vi "首页.vi"() -> ()   [LabVIEW 2016]
uses:
  <vilib>/Utility/miscctls.llb/LVPointTypeDef.ctl
  <vilib>/Utility/sysdir.llb/System Directory Type.ctl
  <vilib>/addons/database/_DB Variant To Data/Database Variant To Data.xnode
  PLC/PLC.lvlib
  <vilib>/ptbypt/NI_PtbyPt.lvlib
panel:
  out "大项目框 17":T1(xcontrol)
  out "大项目框 16":T1(xcontrol)
  out "大项目框 15":T1(xcontrol)
  out "大项目框 14":T1(xcontrol)
  out "大项目框 13":T1(xcontrol)
  in  "左箭头":bool
  in  "右箭头":bool
  out "大项目框 12":T1(xcontrol)
  out "大项目框 11":T1(xcontrol)
  out "大项目框 10":T1(xcontrol)
  out "大项目框 9":T1(xcontrol)
  out "大项目框 8":T1(xcontrol)
  out "大项目框 7":T1(xcontrol)
  out "大项目框 6":T1(xcontrol)
  out "大项目框 5":T1(xcontrol)
  out "大项目框 4":T1(xcontrol)
  out "大项目框 3":T1(xcontrol)
  out "大项目框 2":T1(xcontrol)
  out "大项目框":T1(xcontrol)
  out "湿度":string="75.5 %"
  out "室温":string="25.8 ℃"
  # "室温:"
  # "湿度:"
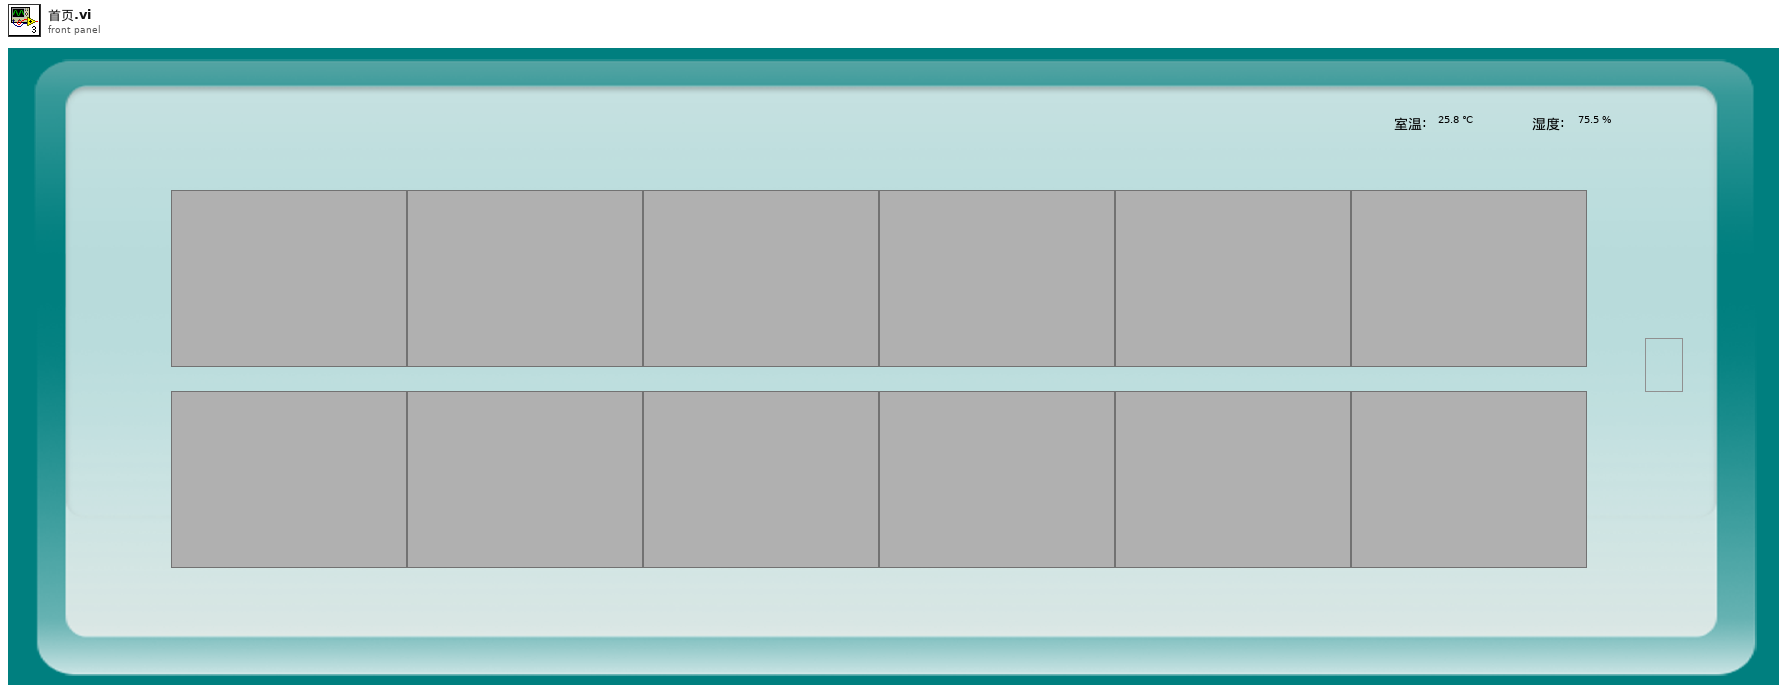
[diagram p1: front panel]
types:
  T1 = cluster{"中文项目名称":string, "英文项目名称":string, "单位":string, "浓度值":string}
  T2 = typedef "LVPointTypeDef.ctl" = cluster{"Horizontal":i16, "Vertical":i16}
  T3 = cluster{"AD0":sgl, "AD1":sgl, "AD2":sgl, "AD3":sgl, "AD4":sgl, "AD5":sgl}
  T4 = typedef "LVDateTimeRec.ctl" = cluster{"秒数的小数部分":dbl, "秒":i32, "分":i32, "时":i32, "日":i32, "月":i32, "年":i32, "天数（周）":i32, "天数（年）":i32, "DST":i32}
  T5 = cluster{"时间标识":timestamp, "监测值":sgl, "单位":string}
  T6 = cluster{"显示参数中文名":string, "显示参数英文名":string, "显示浓度":string, "显示单位":string}[]
  T7 = cluster{"显示参数中文名":string, "显示参数英文名":string, "显示浓度":string, "显示单位":string}
  T8 = typedef "System Directory Type.ctl" = i32
  T9 = cluster{"水温":bool, "pH":bool, "DO":bool, "Cond":bool, "Turb":bool, "氨氮":bool, "总磷":bool, "总氮":bool, "CODMn":bool, "CODCr":bool, "水位":bool, "流速":bool, "瞬时流量":bool, "室温":bool, "湿度":bool, "叶绿素a":bool, "藻密度":bool}
  T10 = cluster{"中文项目名称":string, "英文项目名称":string, "浓度值":string, "单位":string}
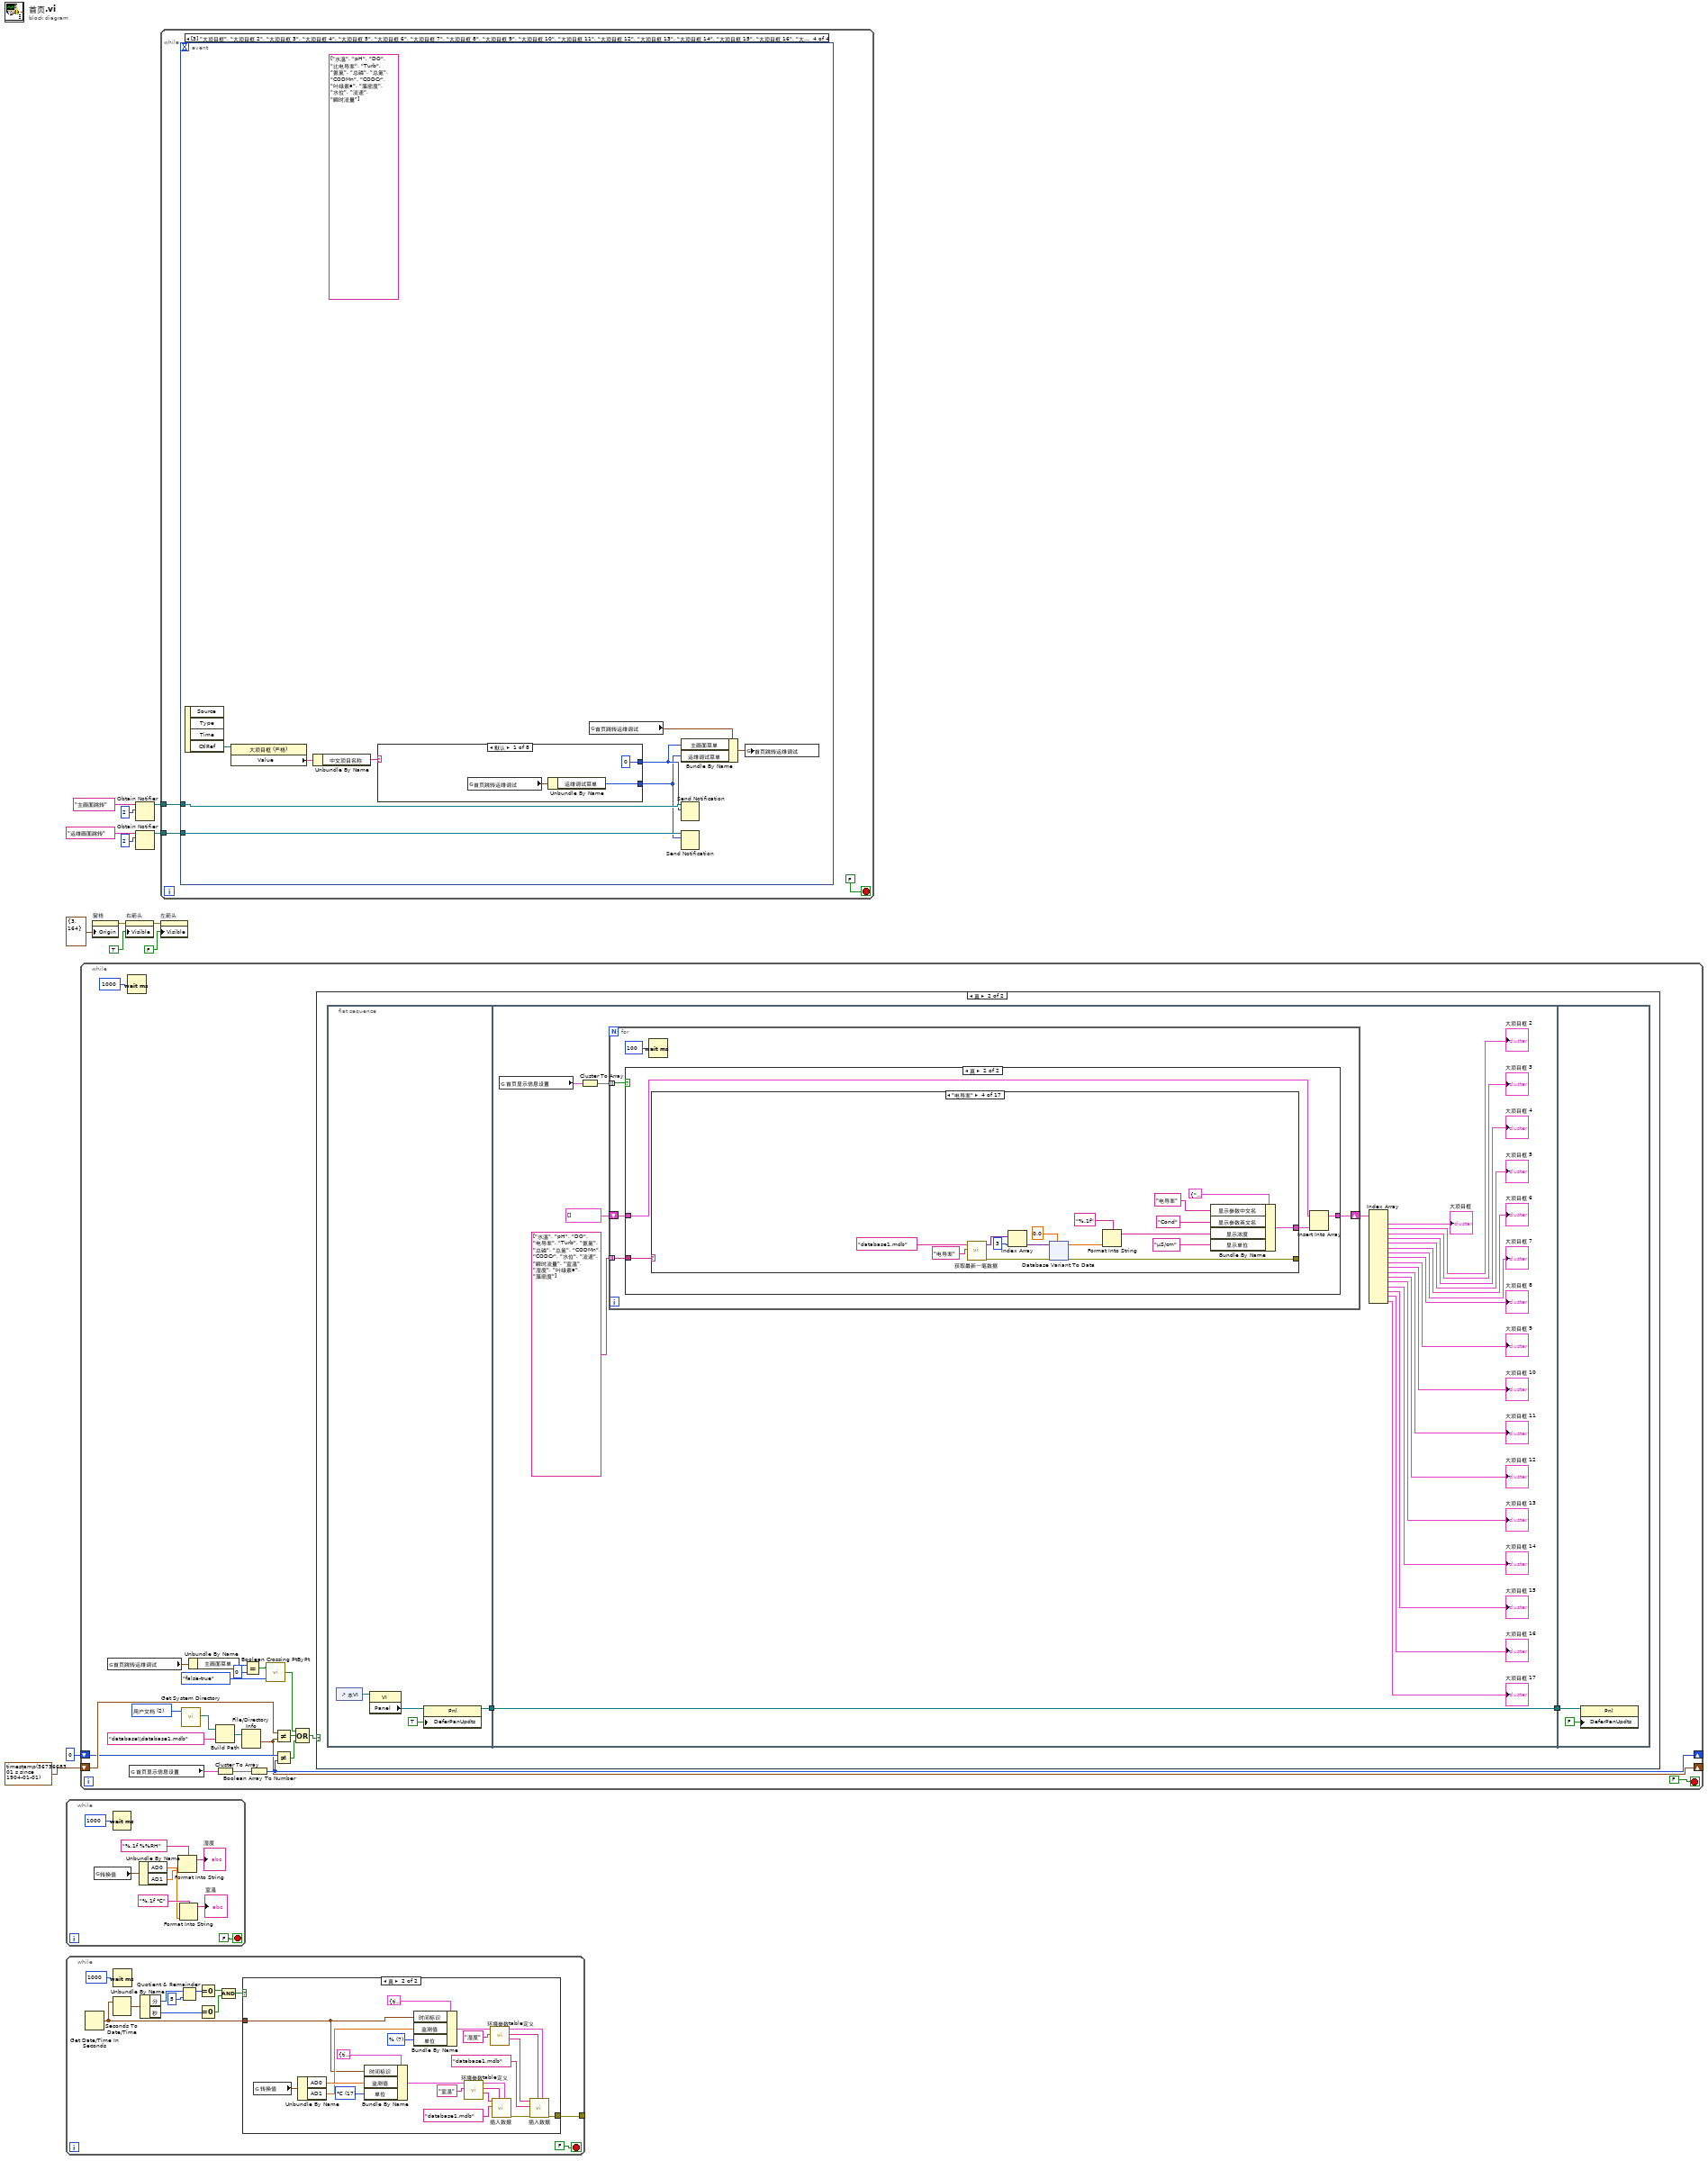
[diagram p0: block diagram]
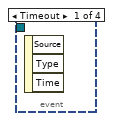
[diagram p3: hidden frame]
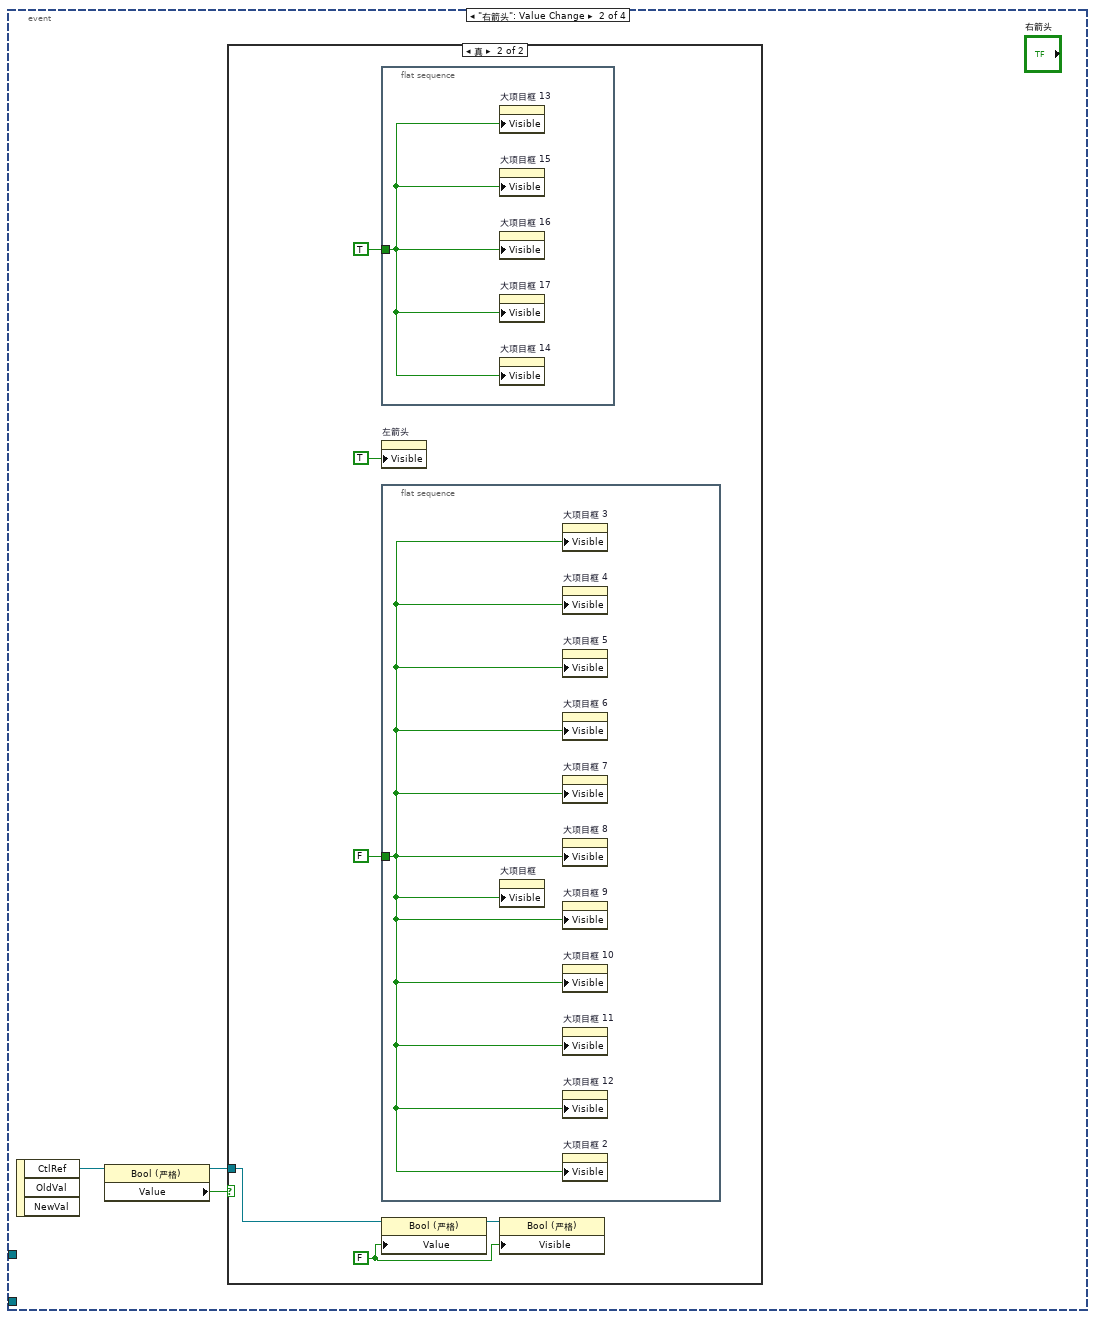
[diagram p4: hidden frame]
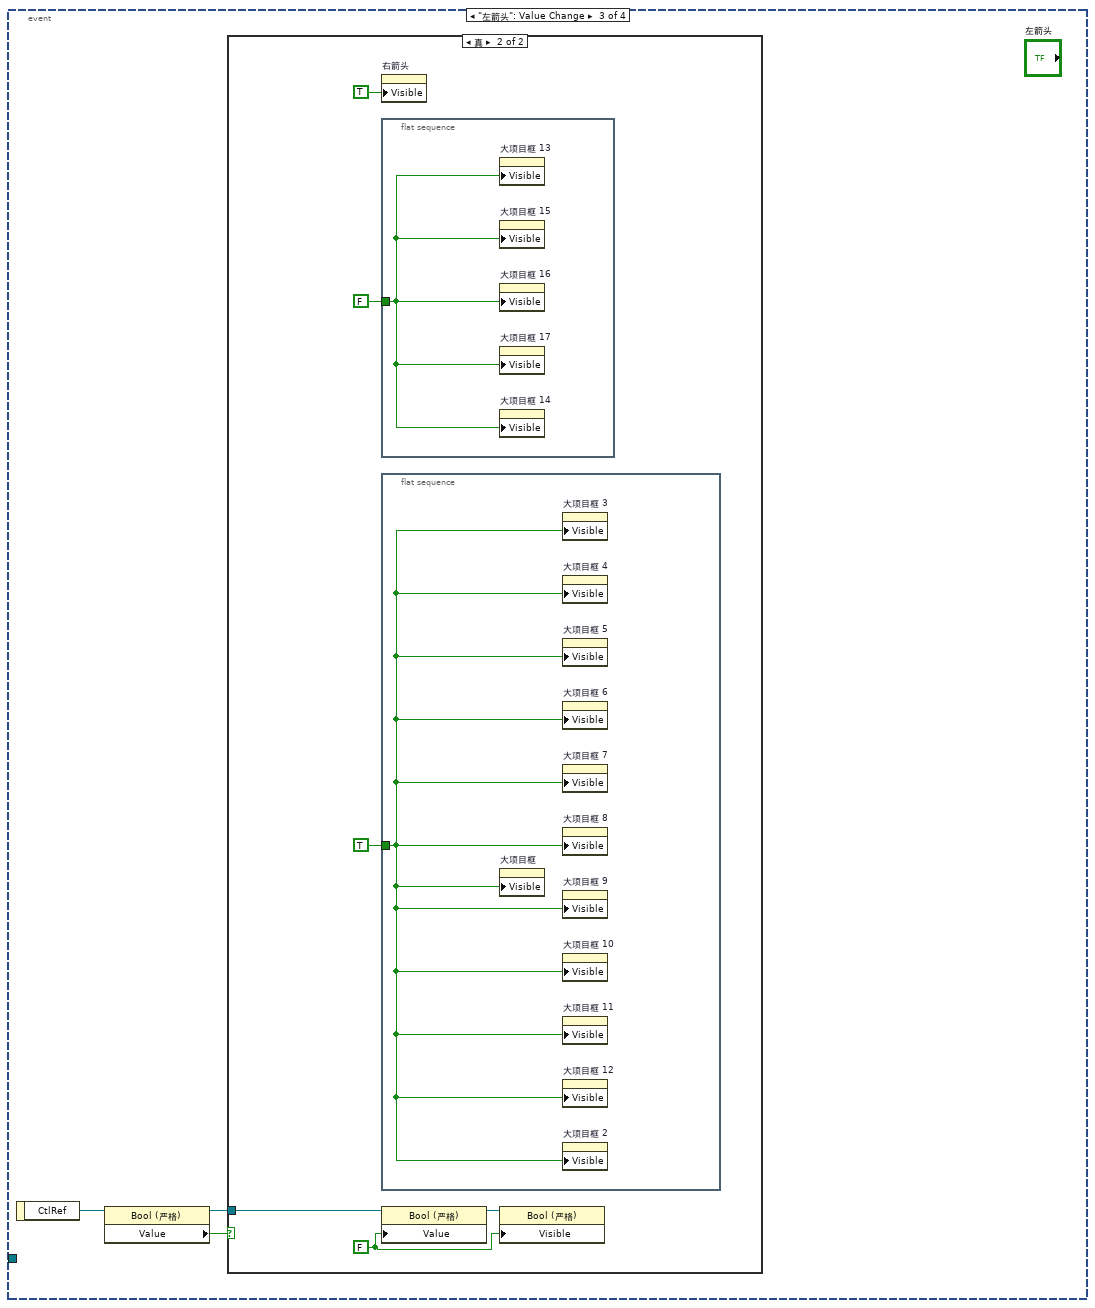
[diagram p6: hidden frame]
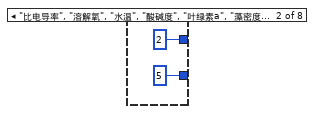
[diagram p8: hidden frame]
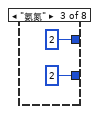
[diagram p9: hidden frame]
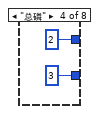
[diagram p10: hidden frame]
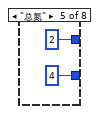
[diagram p11: hidden frame]
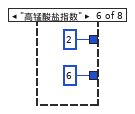
[diagram p12: hidden frame]
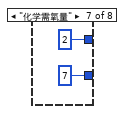
[diagram p13: hidden frame]
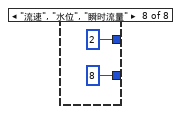
[diagram p14: hidden frame]
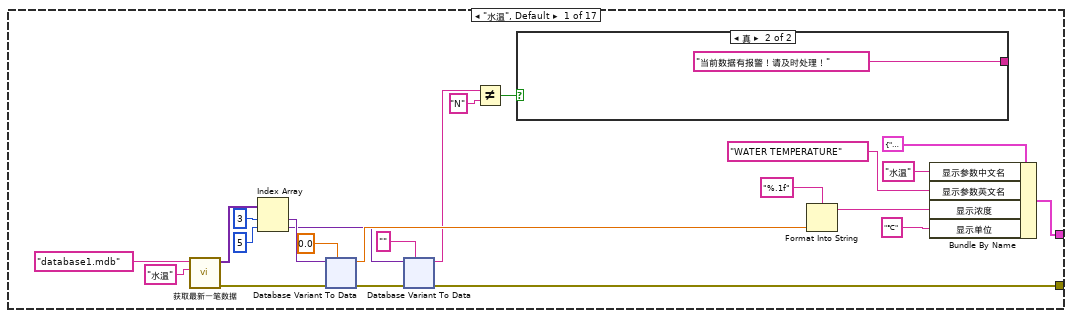
[diagram p17: hidden frame]
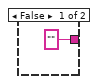
[diagram p18: hidden frame]
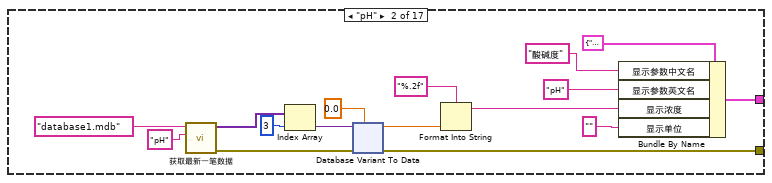
[diagram p19: hidden frame]
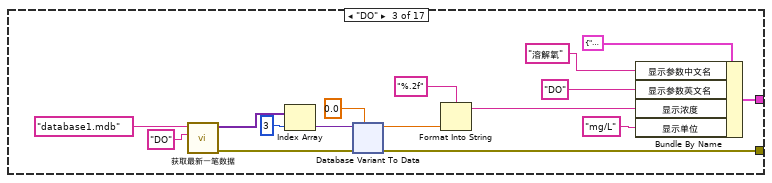
[diagram p20: hidden frame]
diagram:
  n1 = while {
    stop <- FALSE stop-if-true
    n2 = global read "采配水全局变量.vi" "转换值"() -> (w20:T3)
    n3 = Wait (ms)(milliseconds to wait=u32 1000 ("等待时间（毫秒）")) -> ()  [unwired: 1 out]
    n4 = Unbundle By Name(w20) -> ("AD0"=w15:sgl, "AD1"=w14:sgl)
    n5 = Format Into String(format string="%.1f %%RH" ("格式字符串"), w14) -> (resulting string=→"湿度":string)  [unwired: 2 in, 1 out]
    n6 = Format Into String(format string="%.1f ℃" ("格式字符串"), w15) -> (resulting string=→"室温":string)  [unwired: 2 in, 1 out]
  }
  n7 = while {
    tunnel: [w33] -> _
    stop <- FALSE stop-if-true
    n8 = Get Date/Time In Seconds() -> (seconds since 1Jan1904=w32:timestamp)
    n9 = Seconds To Date/Time(time stamp (now)=w32) -> (date time rec=w31:T4)  [unwired: 1 in]
    n10 = Wait (ms)(milliseconds to wait=u32 1000 ("等待时间（毫秒）")) -> ()  [unwired: 1 out]
    n11 = Unbundle By Name(w31) -> ("分"=w30:i32, "秒"=w28:i32)
    n12 = Quotient & Remainder(x=w30, y=5) -> (x-y*floor(x/y)=w27:i32)  [unwired: 1 out]
    n13 = Equal To 0?(x=w27) -> (x = 0?=w26:bool)
    n14 = Equal To 0?(x=w28) -> (x = 0?=w25:bool)
    n15 = Compound Arithmetic op=AND ("复合运算")(w26, w25) -> (w24:bool)
    n16 = case shown="真" w24 {
      tunnel: [_ w48] -> w33
      tunnel: w32 -> [_ w36]
      frame False {
      }
      frame True {
        w41 = u16 7 items=["ug/L", "mg/L", "ppm", "mg/m3", "cm", "ppb", "ug/m3", "%", "nmol/mol", "umol/mol", "MPN/L", "MPN/100ml", "ng/m3", "NTU", "无量纲", "ms/cm", "us/cm", "℃", "V"] ("单位")
        w45 = u16 17 items=["ug/L", "mg/L", "ppm", "mg/m3", "cm", "ppb", "ug/m3", "%", "nmol/mol", "umol/mol", "MPN/L", "MPN/100ml", "ng/m3", "NTU", "无量纲", "ms/cm", "us/cm", "℃", "V"] ("单位")
        n17 = global read "采配水全局变量.vi" "转换值"() -> (w56:T3)
        n18 = Unbundle By Name(w56) -> ("AD0"=w44:sgl, "AD1"=w42:sgl)
        n19 = Bundle By Name(cluster=cluster{"时间标识":timestamp, "监测值":sgl, "单位":u16} {"时间标识"=timestamp(0 s since 1904-01-01), "监测值"=0.0, "单位"=0} ("data"), "时间标识"=w36, "监测值"=w44, "单位"=w45) -> (w46:cluster{"时间标识":timestamp, "监测值":sgl, "单位":u16})
        n20 = Bundle By Name(cluster=cluster{"时间标识":timestamp, "监测值":sgl, "单位":u16} {"时间标识"=timestamp(0 s since 1904-01-01), "监测值"=0.0, "单位"=0} ("data"), "时间标识"=w36, "监测值"=w42, "单位"=w41) -> (w40:cluster{"时间标识":timestamp, "监测值":sgl, "单位":u16})
        n21 = call "环境参数table定义.vi"("table 输入"="室温", "data"=w46) -> ("table 输出"=w55:string, "columns"=w54:string[], "data输出"=w53:T5)  [unwired: 7 in]
        n22 = call "环境参数table定义.vi"("table 输入"="湿度", "data"=w40) -> ("table 输出"=w50:string, "columns"=w51:string[], "data输出"=w52:T5)  [unwired: 7 in]
        n23 = call "插入数据.vi"("data"=w53, "columns"=w54, "database"="database1.mdb" ("table 输入"), "table"=w55) -> ("error out"=w49:errorcluster)  [unwired: 7 in]
        n24 = call "插入数据.vi"("data"=w52, "columns"=w51, "error in (no error)"=w49, "database"="database1.mdb" ("table 输入"), "table"=w50) -> ("error out"=w48:errorcluster)  [unwired: 6 in]
      }
    }
  }
  n25 = while {
    shift-right: [w63] -> _
    shift-left: timestamp(3673668301 s since 1904-01-01) ("上次修改") -> [w72]
    shift-right: [w65] -> _
    shift-left: u32 0 ("数字") -> [w67]
    stop <- FALSE stop-if-true
    w75 = T8 2 items=["用户目录"=0, "用户桌面"=1, "用户文档"=2, "用户应用程序数据"=3, "用户设置"=4, "用户临时目录"=5, "公共文档"=6, "公共应用程序数据"=7, "公共设置"=8, "公共缓存"=13, "系统核心库"=9, "系统安装库"=10, "应用程序文件"=11, "启动盘根目录"=12] ("system directory type")
    n26 = global read "系统设置全局变量.vi" "首页跳转运维调试"() -> (w62:cluster{"主画面菜单":i32, "运维调试菜单":i32})
    n27 = Wait (ms)(milliseconds to wait=u32 1000 ("等待时间（毫秒）")) -> ()  [unwired: 1 out]
    n28 = global read "系统设置全局变量.vi" "首页显示信息设置"() -> (w69:T9)
    n29 = call <vilib>:"Get System Directory.vi"("system directory type"=w75) -> ("system directory"=w74:path)  [unwired: 10 in]
    n30 = Unbundle By Name(w62) -> ("主画面菜单"=w61:i32)
    n31 = Build Path(base path=w74, name or relative path="database\\database1.mdb" ("名称或相对路径")) -> (appended path=w64:path)
    n32 = Cluster To Array(cluster=w69) -> (array=w68:bool[])
    n33 = File/Directory Info(path=w64) -> (last mod=w63:timestamp)  [unwired: 1 in, 6 out]
    n34 = Equal?(x=w61, y=0) -> (x = y?=w59:bool)
    n35 = Boolean Array To Number(Boolean array=w68) -> (number=w65:u32)
    n36 = call <vilib>:"Boolean Crossing PtByPt.vi"("direction"=enum16{"either", "false-true", "true-false"}."false-true", "input"=w59) -> ("crossing"=w57:bool)  [unwired: 1 in]
    n37 = Not Equal?(x=w72, y=w63) -> (x != y?=w71:bool)
    n38 = Not Equal?(x=w67, y=w65) -> (x != y?=w66:bool)
    n39 = Compound Arithmetic op=OR ("复合运算")(w57, w71, w66) -> (w70:bool)
    n40 = case shown="真" w70 {
      frame False {
      }
      frame True {
        n41 = flat-sequence {
          tunnel: [w80] -> w78
          tunnel: [w84] -> w79
          tunnel: w78 -> [w84]
          tunnel: w79 -> [w777]
          frame #0 {
            n42 = control-ref of="本VI"() -> (w81:refnum<vi>)
            n43 = property class="VI"(reference=w81) -> ("Panel"=w82:refnum<vi>)  [unwired: 1 in, 2 out]
            n44 = property class="Pnl"(reference=w82, "DeferPanUpdts"=TRUE ("延迟前面板更新")) -> (reference out=w80:refnum<vi>)  [unwired: 1 in, 1 out]
          }
          frame #1 {
            n45 = global read "系统设置全局变量.vi" "首页显示信息设置"() -> (w86:T9)
            n46 = Cluster To Array(cluster=w86) -> (array=w85:bool[])
            n47 = for {
              tunnel: w85 -> [w111] mode=indexing
              tunnel: string[] ["水温", "pH", "DO", "电导率", "Turb", "氨氮", "总磷", "总氮", "CODMn", "CODCr", "水位", "流速", "瞬时流量", "室温", "湿度", "叶绿素a", "藻密度"] -> [w110] mode=indexing
              shift-right: [w108] -> w106
              shift-left: T6 [] -> [w109]
              n48 = case shown="真" w111 {
                tunnel: w110 -> [_ w116]
                tunnel: w109 -> [w112 w115]
                tunnel: [w112 w114] -> w108
                frame False {
                }
                frame True {
                  n49 = case shown="\"电导率\"" w116 {
                    tunnel: [w125 w217 w265 w313 w361 w409 w457 w505 w553 w601 w639 w687 w737 w745 w750 w760 w769] -> w113
                    tunnel: [w117 w206 w254 w302 w350 w398 w446 w494 w542 w590 w638 w686 _ _ _ _ _] -> _
                    frame "水温", Default {
                      n50 = call "获取最新一笔数据.vi"("table"="水温", "database"="database1.mdb" ("名称或相对路径")) -> ("error out"=w126:errorcluster, "子数组"=w132:variant[])  [unwired: 8 in]
                      n51 = Index Array(array=w132, index #1=3 ("索引"), index #2=5 ("索引")) -> (element #1=w130:variant, element #2=w122:variant)
                      n52 = xnode "Database Variant To Data"("database variant"=w130, "error in (no error)"=w126, "type"=0.0) -> ("data"=w127:dbl, "error out"=w118:errorcluster)
                      n53 = xnode "Database Variant To Data"("database variant"=w122, "error in (no error)"=w118, "type"="") -> ("data"=w121:string, "error out"=w117:errorcluster)
                      n54 = Not Equal?(x=w121, y="N") -> (x != y?=w119:bool)
                      n55 = case shown="真" w119 {
                        tunnel: ["" "当前数据有报警！请及时处理！" ("y")] -> _
                        frame False {
                        }
                        frame True {
                        }
                      }
                      n56 = Format Into String(format string="%.1f" ("格式字符串"), w127) -> (resulting string=w134:string)  [unwired: 2 in, 1 out]
                      n57 = Bundle By Name(cluster=T7 {"显示参数中文名"="", "显示参数英文名"="", "显示浓度"="", "显示单位"=""} ("元素"), "显示参数中文名"="水温", "显示参数英文名"="WATER TEMPERATURE", "显示浓度"=w134, "显示单位"="℃") -> (w125:T7)
                    }
                    frame "pH" {
                      n58 = call "获取最新一笔数据.vi"("table"="pH", "database"="database1.mdb" ("名称或相对路径")) -> ("error out"=w207:errorcluster, "子数组"=w213:variant[])  [unwired: 8 in]
                      n59 = Index Array(array=w213, index=3 ("索引")) -> (element=w211:variant)
                      n60 = xnode "Database Variant To Data"("database variant"=w211, "error in (no error)"=w207, "type"=0.0) -> ("data"=w208:dbl, "error out"=w206:errorcluster)
                      n61 = Format Into String(format string="%.2f" ("格式字符串"), w208) -> (resulting string=w215:string)  [unwired: 2 in, 1 out]
                      n62 = Bundle By Name(cluster=T7 {"显示参数中文名"="", "显示参数英文名"="", "显示浓度"="", "显示单位"=""} ("元素"), "显示参数中文名"="酸碱度", "显示参数英文名"="pH", "显示浓度"=w215, "显示单位"="") -> (w217:T7)
                    }
                    frame "DO" {
                      n63 = call "获取最新一笔数据.vi"("table"="DO", "database"="database1.mdb" ("名称或相对路径")) -> ("error out"=w255:errorcluster, "子数组"=w261:variant[])  [unwired: 8 in]
                      n64 = Index Array(array=w261, index=3 ("索引")) -> (element=w259:variant)
                      n65 = xnode "Database Variant To Data"("database variant"=w259, "error in (no error)"=w255, "type"=0.0) -> ("data"=w256:dbl, "error out"=w254:errorcluster)
                      n66 = Format Into String(format string="%.2f" ("格式字符串"), w256) -> (resulting string=w263:string)  [unwired: 2 in, 1 out]
                      n67 = Bundle By Name(cluster=T7 {"显示参数中文名"="", "显示参数英文名"="", "显示浓度"="", "显示单位"=""} ("元素"), "显示参数中文名"="溶解氧", "显示参数英文名"="DO", "显示浓度"=w263, "显示单位"="mg/L") -> (w265:T7)
                    }
                    frame "电导率" {
                      n68 = call "获取最新一笔数据.vi"("table"="电导率", "database"="database1.mdb" ("名称或相对路径")) -> ("error out"=w303:errorcluster, "子数组"=w309:variant[])  [unwired: 8 in]
                      n69 = Index Array(array=w309, index=3 ("索引")) -> (element=w307:variant)
                      n70 = xnode "Database Variant To Data"("database variant"=w307, "error in (no error)"=w303, "type"=0.0) -> ("data"=w304:dbl, "error out"=w302:errorcluster)
                      n71 = Format Into String(format string="%.1f" ("格式字符串"), w304) -> (resulting string=w311:string)  [unwired: 2 in, 1 out]
                      n72 = Bundle By Name(cluster=T7 {"显示参数中文名"="", "显示参数英文名"="", "显示浓度"="", "显示单位"=""} ("元素"), "显示参数中文名"="电导率", "显示参数英文名"="Cond", "显示浓度"=w311, "显示单位"="μS/cm") -> (w313:T7)
                    }
                    frame "Turb" {
                      n73 = call "获取最新一笔数据.vi"("table"="浊度", "database"="database1.mdb" ("名称或相对路径")) -> ("error out"=w351:errorcluster, "子数组"=w357:variant[])  [unwired: 8 in]
                      n74 = Index Array(array=w357, index=3 ("索引")) -> (element=w355:variant)
                      n75 = xnode "Database Variant To Data"("database variant"=w355, "error in (no error)"=w351, "type"=0.0) -> ("data"=w352:dbl, "error out"=w350:errorcluster)
                      n76 = Format Into String(format string="%.1f" ("格式字符串"), w352) -> (resulting string=w359:string)  [unwired: 2 in, 1 out]
                      n77 = Bundle By Name(cluster=T7 {"显示参数中文名"="", "显示参数英文名"="", "显示浓度"="", "显示单位"=""} ("元素"), "显示参数中文名"="浊度", "显示参数英文名"="Turb", "显示浓度"=w359, "显示单位"="NTU") -> (w361:T7)
                    }
                    frame "氨氮" {
                      n78 = call "获取最新一笔数据.vi"("table"="氨氮", "database"="database1.mdb" ("名称或相对路径")) -> ("error out"=w399:errorcluster, "子数组"=w405:variant[])  [unwired: 8 in]
                      n79 = Index Array(array=w405, index=3 ("索引")) -> (element=w403:variant)
                      n80 = xnode "Database Variant To Data"("database variant"=w403, "error in (no error)"=w399, "type"=0.0) -> ("data"=w400:dbl, "error out"=w398:errorcluster)
                      n81 = Format Into String(format string="%.3f" ("格式字符串"), w400) -> (resulting string=w407:string)  [unwired: 2 in, 1 out]
                      n82 = Bundle By Name(cluster=T7 {"显示参数中文名"="", "显示参数英文名"="", "显示浓度"="", "显示单位"=""} ("元素"), "显示参数中文名"="氨氮", "显示参数英文名"="NPA", "显示浓度"=w407, "显示单位"="mg/L") -> (w409:T7)
                    }
                    frame "总磷" {
                      n83 = call "获取最新一笔数据.vi"("table"="总磷", "database"="database1.mdb" ("名称或相对路径")) -> ("error out"=w447:errorcluster, "子数组"=w453:variant[])  [unwired: 8 in]
                      n84 = Index Array(array=w453, index=3 ("索引")) -> (element=w451:variant)
                      n85 = xnode "Database Variant To Data"("database variant"=w451, "error in (no error)"=w447, "type"=0.0) -> ("data"=w448:dbl, "error out"=w446:errorcluster)
                      n86 = Format Into String(format string="%.3f" ("格式字符串"), w448) -> (resulting string=w455:string)  [unwired: 2 in, 1 out]
                      n87 = Bundle By Name(cluster=T7 {"显示参数中文名"="", "显示参数英文名"="", "显示浓度"="", "显示单位"=""} ("元素"), "显示参数中文名"="总磷", "显示参数英文名"="TP", "显示浓度"=w455, "显示单位"="mg/L") -> (w457:T7)
                    }
                    frame "总氮" {
                      n88 = call "获取最新一笔数据.vi"("table"="总氮", "database"="database1.mdb" ("名称或相对路径")) -> ("error out"=w495:errorcluster, "子数组"=w501:variant[])  [unwired: 8 in]
                      n89 = Index Array(array=w501, index=3 ("索引")) -> (element=w499:variant)
                      n90 = xnode "Database Variant To Data"("database variant"=w499, "error in (no error)"=w495, "type"=0.0) -> ("data"=w496:dbl, "error out"=w494:errorcluster)
                      n91 = Format Into String(format string="%.2f" ("格式字符串"), w496) -> (resulting string=w503:string)  [unwired: 2 in, 1 out]
                      n92 = Bundle By Name(cluster=T7 {"显示参数中文名"="", "显示参数英文名"="", "显示浓度"="", "显示单位"=""} ("元素"), "显示参数中文名"="总氮", "显示参数英文名"="TN", "显示浓度"=w503, "显示单位"="mg/L") -> (w505:T7)
                    }
                    frame "CODMn" {
                      n93 = call "获取最新一笔数据.vi"("table"="CODmn", "database"="database1.mdb" ("名称或相对路径")) -> ("error out"=w543:errorcluster, "子数组"=w549:variant[])  [unwired: 8 in]
                      n94 = Index Array(array=w549, index=3 ("索引")) -> (element=w547:variant)
                      n95 = xnode "Database Variant To Data"("database variant"=w547, "error in (no error)"=w543, "type"=0.0) -> ("data"=w544:dbl, "error out"=w542:errorcluster)
                      n96 = Format Into String(format string="%.2f" ("格式字符串"), w544) -> (resulting string=w551:string)  [unwired: 2 in, 1 out]
                      n97 = Bundle By Name(cluster=T7 {"显示参数中文名"="", "显示参数英文名"="", "显示浓度"="", "显示单位"=""} ("元素"), "显示参数中文名"="高锰酸盐指数", "显示参数英文名"="CODmn", "显示浓度"=w551, "显示单位"="mg/L") -> (w553:T7)
                    }
                    frame "CODCr" {
                      n98 = call "获取最新一笔数据.vi"("table"="CODCr", "database"="database1.mdb" ("名称或相对路径")) -> ("error out"=w591:errorcluster, "子数组"=w597:variant[])  [unwired: 8 in]
                      n99 = Index Array(array=w597, index=3 ("索引")) -> (element=w595:variant)
                      n100 = xnode "Database Variant To Data"("database variant"=w595, "error in (no error)"=w591, "type"=0.0) -> ("data"=w592:dbl, "error out"=w590:errorcluster)
                      n101 = Format Into String(format string="%.2f" ("格式字符串"), w592) -> (resulting string=w599:string)  [unwired: 2 in, 1 out]
                      n102 = Bundle By Name(cluster=T7 {"显示参数中文名"="", "显示参数英文名"="", "显示浓度"="", "显示单位"=""} ("元素"), "显示参数中文名"="化学需氧量", "显示参数英文名"="CODCr", "显示浓度"=w599, "显示单位"="mg/L") -> (w601:T7)
                    }
                    frame "叶绿素a" {
                      n103 = call "获取最新一笔数据.vi"("table"="叶绿素a", "database"="database1.mdb" ("名称或相对路径")) -> ("error out"=w640:errorcluster, "子数组"=w646:variant[])  [unwired: 8 in]
                      n104 = Index Array(array=w646, index=3 ("索引")) -> (element=w644:variant)
                      n105 = xnode "Database Variant To Data"("database variant"=w644, "error in (no error)"=w640, "type"=0.0) -> ("data"=w641:dbl, "error out"=w638:errorcluster)
                      n106 = Format Into String(format string="%.2f" ("格式字符串"), w641) -> (resulting string=w648:string)  [unwired: 2 in, 1 out]
                      n107 = Bundle By Name(cluster=T7 {"显示参数中文名"="", "显示参数英文名"="", "显示浓度"="", "显示单位"=""} ("元素"), "显示参数中文名"="叶绿素a", "显示参数英文名"="Chla", "显示浓度"=w648, "显示单位"="μg/L") -> (w639:T7)
                    }
                    frame "藻密度" {
                      n108 = call "获取最新一笔数据.vi"("table"="藻密度", "database"="database1.mdb" ("名称或相对路径")) -> ("error out"=w688:errorcluster, "子数组"=w694:variant[])  [unwired: 8 in]
                      n109 = Index Array(array=w694, index=3 ("索引")) -> (element=w692:variant)
                      n110 = xnode "Database Variant To Data"("database variant"=w692, "error in (no error)"=w688, "type"=0.0) -> ("data"=w689:dbl, "error out"=w686:errorcluster)
                      n111 = Format Into String(format string="%.2f" ("格式字符串"), w689) -> (resulting string=w696:string)  [unwired: 2 in, 1 out]
                      n112 = Bundle By Name(cluster=T7 {"显示参数中文名"="", "显示参数英文名"="", "显示浓度"="", "显示单位"=""} ("元素"), "显示参数中文名"="藻密度", "显示参数英文名"="Algal", "显示浓度"=w696, "显示单位"="cells/mL") -> (w687:T7)
                    }
                    frame "水位" {
                      n113 = global read "流量计全局变量.vi" "水位"() -> (w734:dbl)
                      n114 = Format Into String(format string="%.2f" ("格式字符串"), w734) -> (resulting string=w735:string)  [unwired: 2 in, 1 out]
                      n115 = Bundle By Name(cluster=T7 {"显示参数中文名"="", "显示参数英文名"="", "显示浓度"="", "显示单位"=""} ("元素"), "显示参数中文名"="水位", "显示参数英文名"="WaterLevel", "显示浓度"=w735, "显示单位"="m") -> (w737:T7)
                    }
                    frame "流速" {
                      n116 = global read "流量计全局变量.vi" "瞬时流速"() -> (w742:dbl)
                      n117 = Format Into String(format string="%.2f" ("格式字符串"), w742) -> (resulting string=w743:string)  [unwired: 2 in, 1 out]
                      n118 = Bundle By Name(cluster=T7 {"显示参数中文名"="", "显示参数英文名"="", "显示浓度"="", "显示单位"=""} ("元素"), "显示参数中文名"="流速", "显示参数英文名"="FlowRate", "显示浓度"=w743, "显示单位"="m/s") -> (w745:T7)
                    }
                    frame "瞬时流量" {
                      n119 = global read "流量计全局变量.vi" "瞬时流量"() -> (w751:dbl)
                      n120 = Format Into String(format string="%.2f" ("格式字符串"), w751) -> (resulting string=w752:string)  [unwired: 2 in, 1 out]
                      n121 = Bundle By Name(cluster=T7 {"显示参数中文名"="", "显示参数英文名"="", "显示浓度"="", "显示单位"=""} ("元素"), "显示参数中文名"="瞬时流量", "显示参数英文名"="InstantaneousFlow", "显示浓度"=w752, "显示单位"="m3/s") -> (w750:T7)
                    }
                    frame "室温" {
                      n122 = global read "采配水全局变量.vi" "转换值"() -> (w759:T3)
                      n123 = Unbundle By Name(w759) -> ("AD0"=w758:sgl)
                      n124 = Format Into String(format string="%.2f" ("格式字符串"), w758) -> (resulting string=w761:string)  [unwired: 2 in, 1 out]
                      n125 = Bundle By Name(cluster=T7 {"显示参数中文名"="", "显示参数英文名"="", "显示浓度"="", "显示单位"=""} ("元素"), "显示参数中文名"="室温", "显示参数英文名"="Room Temperature ", "显示浓度"=w761, "显示单位"="℃") -> (w760:T7)
                    }
                    frame "湿度" {
                      n126 = global read "采配水全局变量.vi" "转换值"() -> (w768:T3)
                      n127 = Unbundle By Name(w768) -> ("AD1"=w767:sgl)
                      n128 = Format Into String(format string="%.2f" ("格式字符串"), w767) -> (resulting string=w770:string)  [unwired: 2 in, 1 out]
                      n129 = Bundle By Name(cluster=T7 {"显示参数中文名"="", "显示参数英文名"="", "显示浓度"="", "显示单位"=""} ("元素"), "显示参数中文名"="相对湿度", "显示参数英文名"="Relative Humidity", "显示浓度"=w770, "显示单位"="%RH") -> (w769:T7)
                    }
                  }
                  n130 = Insert Into Array(array=w115, new element=w113) -> (w114:T6)  [unwired: 1 in]
                }
              }
              n131 = Wait (ms)(milliseconds to wait=u32 100 ("等待时间（毫秒）")) -> ()  [unwired: 1 out]
            }
            n132 = Index Array(array=w106) -> (element #1=→"大项目框":T7, element #2=→"大项目框 2":T7, element #3=→"大项目框 3":T7, element #4=→"大项目框 4":T7, element #5=→"大项目框 5":T7, element #6=→"大项目框 6":T7, element #7=→"大项目框 7":T7, element #8=→"大项目框 8":T7, element #9=→"大项目框 9":T7, element #10=→"大项目框 10":T7, element #11=→"大项目框 11":T7, element #12=→"大项目框 12":T7, element #13=→"大项目框 13":T7, element #14=→"大项目框 14":T7, element #15=→"大项目框 15":T7, element #16=→"大项目框 16":T7, element #17=→"大项目框 17":T7)  [unwired: 17 in]
          }
          frame #2 {
            n133 = property class="Pnl"(reference=w777, "DeferPanUpdts"=FALSE ("延迟前面板更新")) -> ()  [unwired: 1 in, 2 out]
          }
        }
      }
    }
  }
  n134 = property on="窗格" class="Pane"("Origin"=T2 {"Horizontal"=3, "Vertical"=164} ("原点")) -> (error out=w10:errorcluster)  [unwired: 2 in, 1 out]
  n135 = property on="右箭头" class="Bool (严格)"(error in=w10, "Visible"=TRUE ("可见")) -> (error out=w9:errorcluster)  [unwired: 1 in, 1 out]
  n136 = Obtain Notifier(name (unnamed)="主画面跳转" ("名称（未命名）"), notification data type=2 ("主画面菜单")) -> (notifier out=w8:refnum<notifier>)  [unwired: 2 in, 2 out]
  n137 = Obtain Notifier(name (unnamed)="运维画面跳转" ("名称（未命名）"), notification data type=2 ("主画面菜单")) -> (notifier out=w3:refnum<notifier>)  [unwired: 2 in, 2 out]
  n138 = property on="左箭头" class="Bool (严格)"(error in=w9, "Visible"=FALSE ("可见")) -> ()  [unwired: 1 in, 2 out]
  n139 = while {
    tunnel: w8 -> [w779]
    tunnel: w3 -> [w778]
    stop <- FALSE stop-if-true
    n140 = event shown="[3] \"大项目框\", \"大项目框 2\", \"大项目框 3\", \"大项目框 4\", \"大项目框 5\", \"大项目框 6\", \"大项目框 7\", \"大项目框 8\", \"大项目框 9\", \"大项目框 10\", \"大项目框 11\", \"大项目框 12\", \"大项目框 13\", \"大项目框 14\", \"大项目框 15\", \"大项目框 16\", \"大项目框 17\": 鼠标按下" {
      selector: _ -> [_ _ _ _]
      dyn-events: _ -> [_ _ _ _]
      timeout: _ -> [_ _ _ _]
      tunnel: w779 -> [_ _ _ w807]
      tunnel: w778 -> [_ _ _ w804]
      event Timeout {
        n141 = event-data() -> ()  [unwired: 1 in, 3 out]
      }
      event "右箭头": Value Change {
        n142 = event-data() -> ("CtlRef"=w783:refnum<vi>)  [unwired: 1 in, 2 out]
        n143 = property class="Bool (严格)"(reference=w783) -> (reference out=w781:refnum<vi>, "Value"=w782:bool)  [unwired: 1 in, 1 out]
        n144 = case shown="真" w782 {
          tunnel: w781 -> [_ w789]
          frame False {
          }
          frame True {
            w788 = FALSE ("值")
            n145 = flat-sequence {
              tunnel: TRUE ("可见") -> [w790]
              frame #0 {
                n146 = property on="大项目框 13" class="大项目框 (严格)"("Visible"=w790) -> ()  [unwired: 2 in, 2 out]
                n147 = property on="大项目框 15" class="大项目框 (严格)"("Visible"=w790) -> ()  [unwired: 2 in, 2 out]
                n148 = property on="大项目框 16" class="大项目框 (严格)"("Visible"=w790) -> ()  [unwired: 2 in, 2 out]
                n149 = property on="大项目框 17" class="大项目框 (严格)"("Visible"=w790) -> ()  [unwired: 2 in, 2 out]
                n150 = property on="大项目框 14" class="大项目框 (严格)"("Visible"=w790) -> ()  [unwired: 2 in, 2 out]
              }
            }
            n151 = property on="左箭头" class="Bool (严格)"("Visible"=TRUE ("可见")) -> ()  [unwired: 2 in, 2 out]
            n152 = flat-sequence {
              tunnel: FALSE ("可见") -> [w791]
              frame #0 {
                n153 = property on="大项目框" class="大项目框 (严格)"("Visible"=w791) -> ()  [unwired: 2 in, 2 out]
                n154 = property on="大项目框 3" class="大项目框 (严格)"("Visible"=w791) -> ()  [unwired: 2 in, 2 out]
                n155 = property on="大项目框 4" class="大项目框 (严格)"("Visible"=w791) -> ()  [unwired: 2 in, 2 out]
                n156 = property on="大项目框 5" class="大项目框 (严格)"("Visible"=w791) -> ()  [unwired: 2 in, 2 out]
                n157 = property on="大项目框 6" class="大项目框 (严格)"("Visible"=w791) -> ()  [unwired: 2 in, 2 out]
                n158 = property on="大项目框 7" class="大项目框 (严格)"("Visible"=w791) -> ()  [unwired: 2 in, 2 out]
                n159 = property on="大项目框 8" class="大项目框 (严格)"("Visible"=w791) -> ()  [unwired: 2 in, 2 out]
                n160 = property on="大项目框 9" class="大项目框 (严格)"("Visible"=w791) -> ()  [unwired: 2 in, 2 out]
                n161 = property on="大项目框 10" class="大项目框 (严格)"("Visible"=w791) -> ()  [unwired: 2 in, 2 out]
                n162 = property on="大项目框 11" class="大项目框 (严格)"("Visible"=w791) -> ()  [unwired: 2 in, 2 out]
                n163 = property on="大项目框 12" class="大项目框 (严格)"("Visible"=w791) -> ()  [unwired: 2 in, 2 out]
                n164 = property on="大项目框 2" class="大项目框 (严格)"("Visible"=w791) -> ()  [unwired: 2 in, 2 out]
              }
            }
            n165 = property class="Bool (严格)"(reference=w789, "Value"=w788) -> (reference out=w787:refnum<vi>)  [unwired: 1 in, 1 out]
            n166 = property class="Bool (严格)"(reference=w787, "Visible"=w788) -> ()  [unwired: 1 in, 2 out]
          }
        }
      }
      event "左箭头": Value Change {
        n167 = event-data() -> ("CtlRef"=w794:refnum<vi>)  [unwired: 1 in]
        n168 = property class="Bool (严格)"(reference=w794) -> (reference out=w792:refnum<vi>, "Value"=w793:bool)  [unwired: 1 in, 1 out]
        n169 = case shown="真" w793 {
          tunnel: w792 -> [_ w800]
          frame False {
          }
          frame True {
            w799 = FALSE ("值")
            n170 = property on="右箭头" class="Bool (严格)"("Visible"=TRUE ("可见")) -> ()  [unwired: 2 in, 2 out]
            n171 = flat-sequence {
              tunnel: FALSE ("可见") -> [w801]
              frame #0 {
                n172 = property on="大项目框 13" class="大项目框 (严格)"("Visible"=w801) -> ()  [unwired: 2 in, 2 out]
                n173 = property on="大项目框 15" class="大项目框 (严格)"("Visible"=w801) -> ()  [unwired: 2 in, 2 out]
                n174 = property on="大项目框 16" class="大项目框 (严格)"("Visible"=w801) -> ()  [unwired: 2 in, 2 out]
                n175 = property on="大项目框 17" class="大项目框 (严格)"("Visible"=w801) -> ()  [unwired: 2 in, 2 out]
                n176 = property on="大项目框 14" class="大项目框 (严格)"("Visible"=w801) -> ()  [unwired: 2 in, 2 out]
              }
            }
            n177 = flat-sequence {
              tunnel: TRUE ("可见") -> [w802]
              frame #0 {
                n178 = property on="大项目框" class="大项目框 (严格)"("Visible"=w802) -> ()  [unwired: 2 in, 2 out]
                n179 = property on="大项目框 3" class="大项目框 (严格)"("Visible"=w802) -> ()  [unwired: 2 in, 2 out]
                n180 = property on="大项目框 4" class="大项目框 (严格)"("Visible"=w802) -> ()  [unwired: 2 in, 2 out]
                n181 = property on="大项目框 5" class="大项目框 (严格)"("Visible"=w802) -> ()  [unwired: 2 in, 2 out]
                n182 = property on="大项目框 6" class="大项目框 (严格)"("Visible"=w802) -> ()  [unwired: 2 in, 2 out]
                n183 = property on="大项目框 7" class="大项目框 (严格)"("Visible"=w802) -> ()  [unwired: 2 in, 2 out]
                n184 = property on="大项目框 8" class="大项目框 (严格)"("Visible"=w802) -> ()  [unwired: 2 in, 2 out]
                n185 = property on="大项目框 9" class="大项目框 (严格)"("Visible"=w802) -> ()  [unwired: 2 in, 2 out]
                n186 = property on="大项目框 10" class="大项目框 (严格)"("Visible"=w802) -> ()  [unwired: 2 in, 2 out]
                n187 = property on="大项目框 11" class="大项目框 (严格)"("Visible"=w802) -> ()  [unwired: 2 in, 2 out]
                n188 = property on="大项目框 12" class="大项目框 (严格)"("Visible"=w802) -> ()  [unwired: 2 in, 2 out]
                n189 = property on="大项目框 2" class="大项目框 (严格)"("Visible"=w802) -> ()  [unwired: 2 in, 2 out]
              }
            }
            n190 = property class="Bool (严格)"(reference=w800, "Value"=w799) -> (reference out=w798:refnum<vi>)  [unwired: 1 in, 1 out]
            n191 = property class="Bool (严格)"(reference=w798, "Visible"=w799) -> ()  [unwired: 1 in, 2 out]
          }
        }
      }
      event "大项目框", "大项目框 2", "大项目框 3", "大项目框 4", "大项目框 5", "大项目框 6", "大项目框 7", "大项目框 8", "大项目框 9", "大项目框 10", "大项目框 11", "大项目框 12", "大项目框 13", "大项目框 14", "大项目框 15", "大项目框 16", "大项目框 17": Mouse Down {
        (unwired) string[] ["水温", "pH", "DO", "比电导率", "Turb", "氨氮", "总磷", "总氮", "CODMn", "CODCr", "叶绿素a", "藻密度", "水位", "流速", "瞬时流量"]
        n192 = event-data() -> ("CtlRef"=w811:refnum<vi>)  [unwired: 1 in, 3 out]
        n193 = property class="大项目框 (严格)"(reference=w811) -> ("Value"=w810:T10)  [unwired: 1 in, 2 out]
        n194 = Unbundle By Name(w810) -> ("中文项目名称"=w809:string)
        n195 = case shown="默认" w809 {
          tunnel: [w813 5 ("运维调试菜单") 2 ("运维调试菜单") 3 ("运维调试菜单") 4 ("运维调试菜单") 6 ("运维调试菜单") 7 ("运维调试菜单") 8 ("运维调试菜单")] -> w803
          tunnel: [0 ("运维调试菜单") 2 ("运维调试菜单") 2 ("运维调试菜单") 2 ("运维调试菜单") 2 ("运维调试菜单") 2 ("运维调试菜单") 2 ("运维调试菜单") 2 ("运维调试菜单")] -> w805
          frame Default {
            n196 = global read "系统设置全局变量.vi" "首页跳转运维调试"() -> (w814:cluster{"主画面菜单":i32, "运维调试菜单":i32})
            n197 = Unbundle By Name(w814) -> ("运维调试菜单"=w813:i32)
          }
          frame "比电导率", "溶解氧", "水温", "酸碱度", "叶绿素a", "藻密度", "浊度" {
          }
          frame "氨氮" {
          }
          frame "总磷" {
          }
          frame "总氮" {
          }
          frame "高锰酸盐指数" {
          }
          frame "化学需氧量" {
          }
          frame "流速", "水位", "瞬时流量" {
          }
        }
        n198 = global read "系统设置全局变量.vi" "首页跳转运维调试"() -> (w808:cluster{"主画面菜单":i32, "运维调试菜单":i32})
        n199 = Bundle By Name(cluster=w808, "主画面菜单"=w805, "运维调试菜单"=w803) -> (w806:cluster{"主画面菜单":i32, "运维调试菜单":i32})
        n200 = Send Notification(notification=w805, notifier=w807) -> ()  [unwired: 1 in, 2 out]
        n201 = Send Notification(notification=w803, notifier=w804) -> ()  [unwired: 1 in, 2 out]
        n202 = global write "系统设置全局变量.vi" "首页跳转运维调试"(w806) -> ()
      }
    }
  }
